vi "CANbus Mngr 1.vi"(5 "DBC File":path=path "C:/Users/ykouchnir/Desktop/Comemso BCS Tester/BCS24_CAN-MatrixV7_12.dbc", 6 "interface":refnum<k21>="CAN1", 7 "Action":T3, 8 "error in (no error)":errorcluster, 9 "Transfer Type":T1, 10 "database alias":string="Database", 11 "Data in":T2[](array[typedef])) -> (0 "error out":errorcluster, 3 "Data out":T2[](array[typedef]))   [LabVIEW 2021]
uses:
  <vilib>/xnet/xnet.llb/XNET Create Session (Signal Input Single-point).vi
  <resource>/objmgr/xnet.rc
  <vilib>/xnet/xnet.llb/XNET Read (Signal Single-point).vi
  <vilib>/xnet/xnet.llb/XNET Write (Frame CAN).vi
  <vilib>/xnet/xnet.llb/XNET Create Session (Frame Output Single-point).vi
  <vilib>/xnet/xnet.llb/XNET Write (Signal Single-point).vi
  <vilib>/xnet/xnet.llb/XNET Create Session (Conversion).vi
  <vilib>/xnet/xnet.llb/XNET Read (Frame CAN).vi
  <vilib>/xnet/xnet.llb/XNET Convert (Signal to Frame CAN).vi
  controls/Signal Data.ctl
  <vilib>/xnet/xnet.llb/XNET Create Session (Frame Input Single-point).vi
  <vilib>/xnet/xnet.llb/XNET Create Session (Signal Output Single-point).vi
  controls/BCS Manager.ctl
  controls/Transfer Type.ctl
panel:
  in  "JSON?":bool
  in  "JSON signals file":path
  in  "timeout":i32=-1
  in  "number to read":i32=-1
  in  "Termination":u32(ring) items=["Off", "On"]
  in  "Baud Rate":u64=1000000
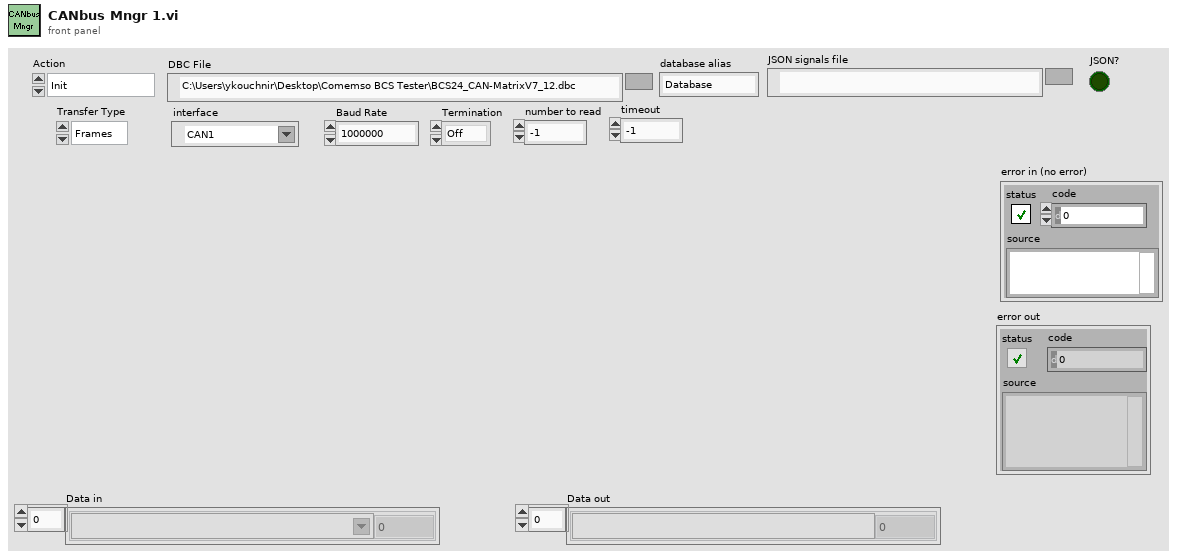
[diagram p1: front panel]
types:
  T1 = typedef "Transfer Type.ctl" = enum16{"Frames", "Signals"}
  T2 = typedef "Signal Data.ctl" = cluster{"XNET Signal":refnum<k21>, "Data":dbl}
  T3 = typedef "BCS Manager.ctl" = enum16{"Init", "Start Signal Session", "Start Frame Session", "Write Sigs Session", "Write Frames Session", "Write Sigs Single", "Write Frames Single", "Read Sigs Session", "Read Frames Session", "Read Sigs Single", "Read Frames Single", "Write Raw Frame Session", "Write Raw Frame Single", "FrameRef to Sigs", "FrameID to FrameRef", "Close"}
  T4 = typedef "JSON sigs.ctl" = cluster{"Read Signals Cyclic":refnum<k21>[], "Write Signals Cyclic":refnum<k21>[], "Write Frames Cyclic":refnum<k21>[], "Read Frames Cyclic":refnum<k21>[], "Write Frames Single":refnum<k21>[], "Read Frames Single":refnum<k21>[], "Write Signals Single":refnum<k21>[], "Read Signals Single":refnum<k21>[]}
  T5 = typedef "XNET Frame CAN.ctl" = cluster{"timestamp":timestamp, "payload":u8[], "identifier":u32, "type":T6, "extended?":bool, "echo?":bool}
  T6 = typedef "XNET Frame Type CAN.ctl" = u8
  T7 = typedef "Frame Data.ctl" = cluster{"Raw Frame":T5, "Frame Name":refnum<k21>, "Signals":T2[]}
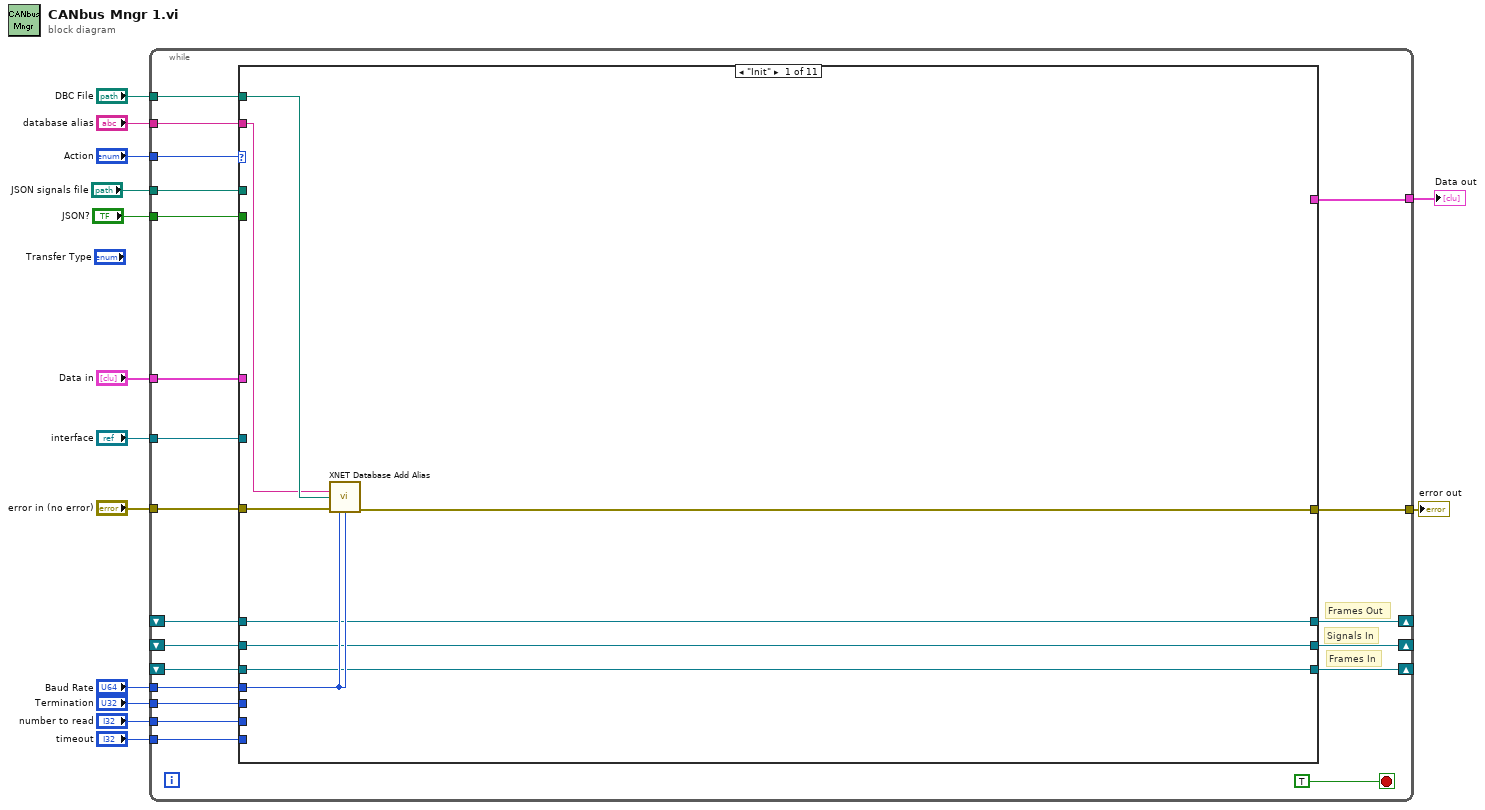
[diagram p0: block diagram]
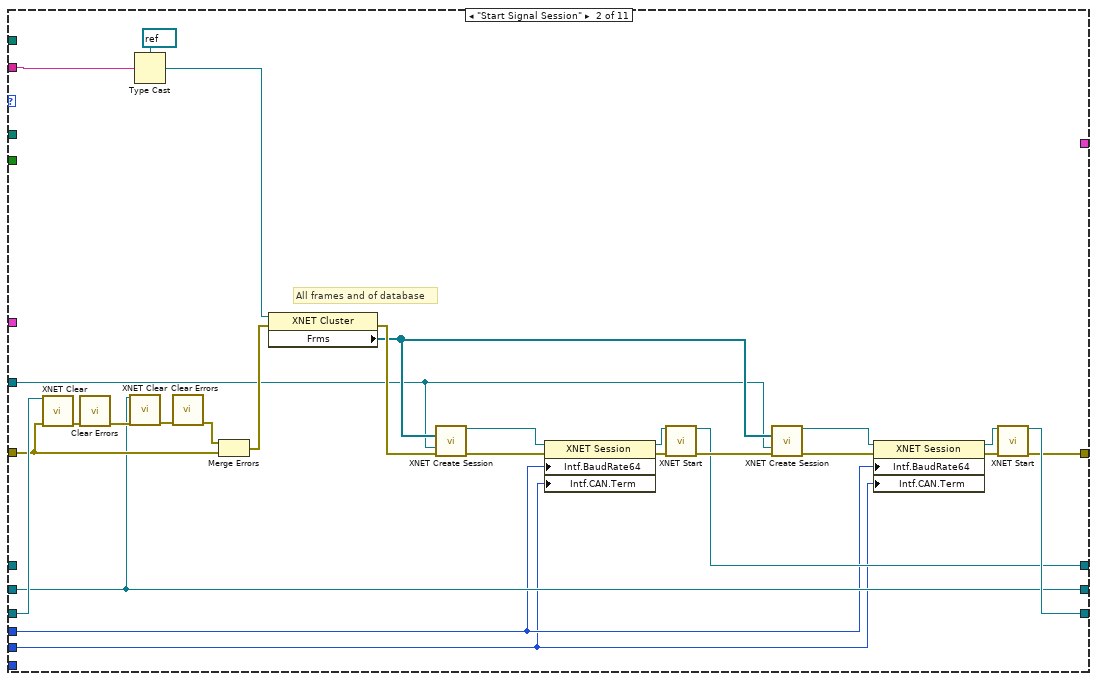
[diagram p2: hidden frame]
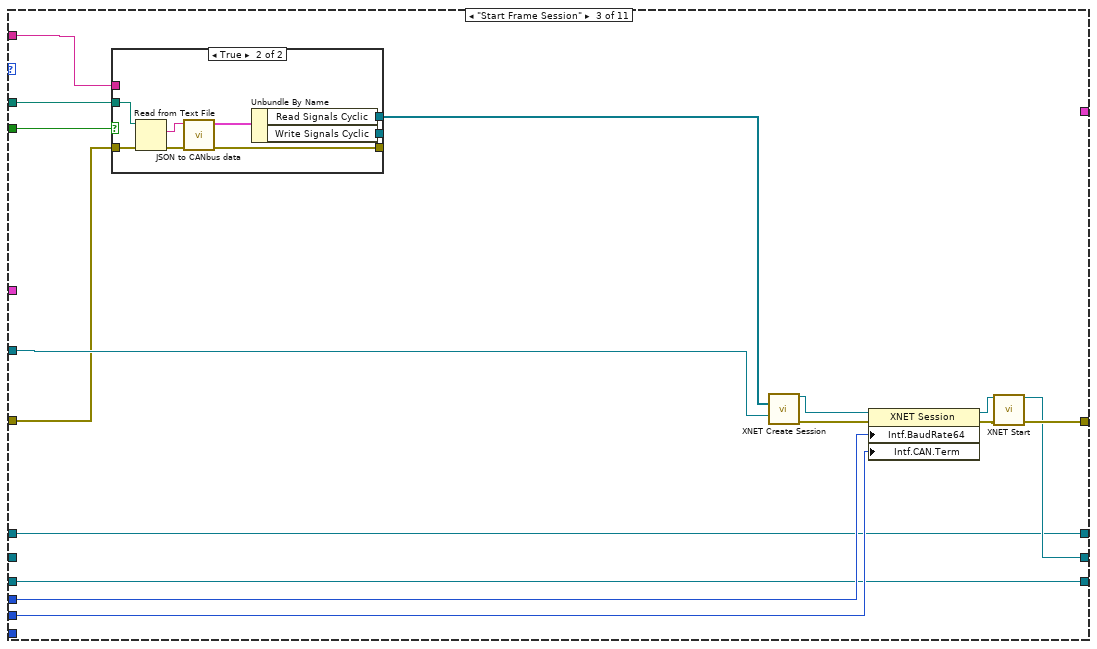
[diagram p3: hidden frame]
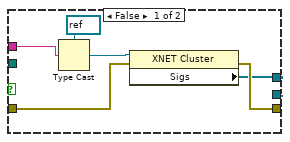
[diagram p4: hidden frame]
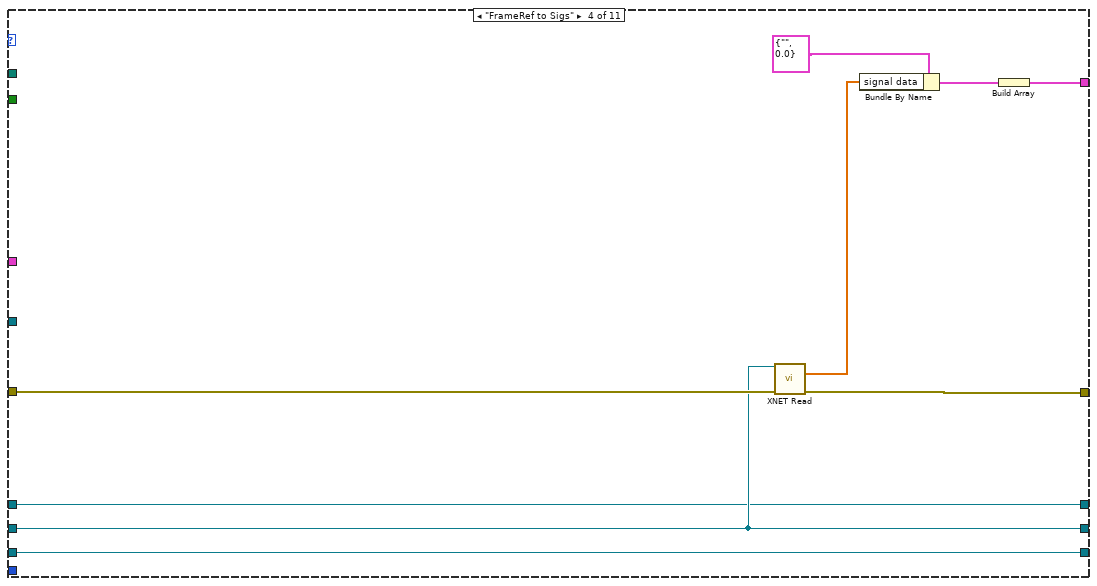
[diagram p5: hidden frame]
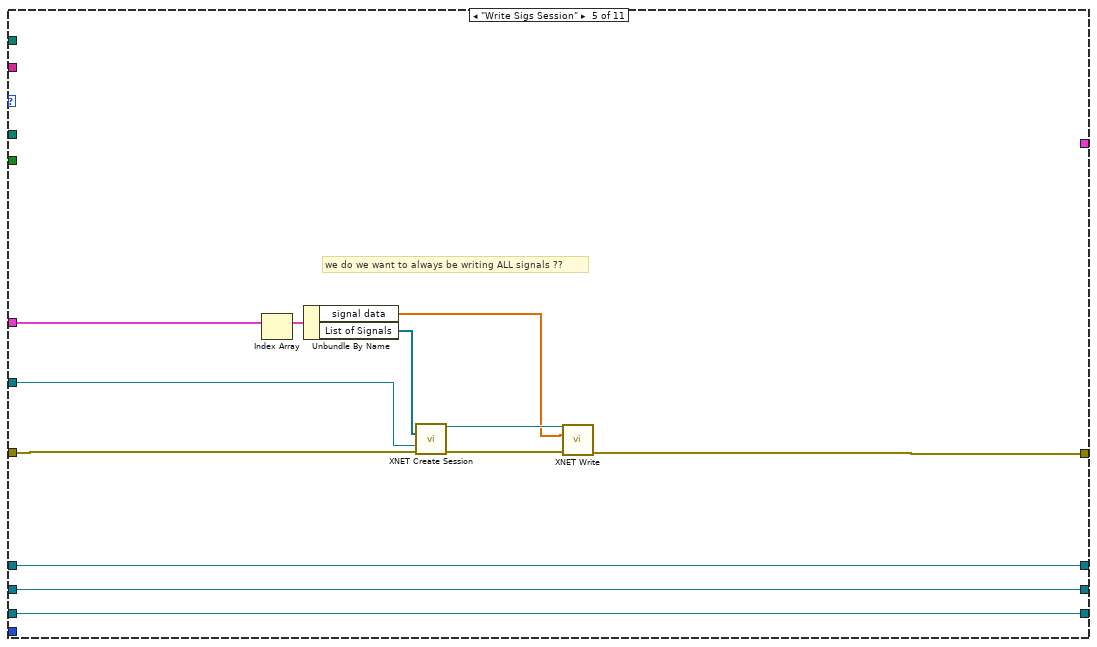
[diagram p6: hidden frame]
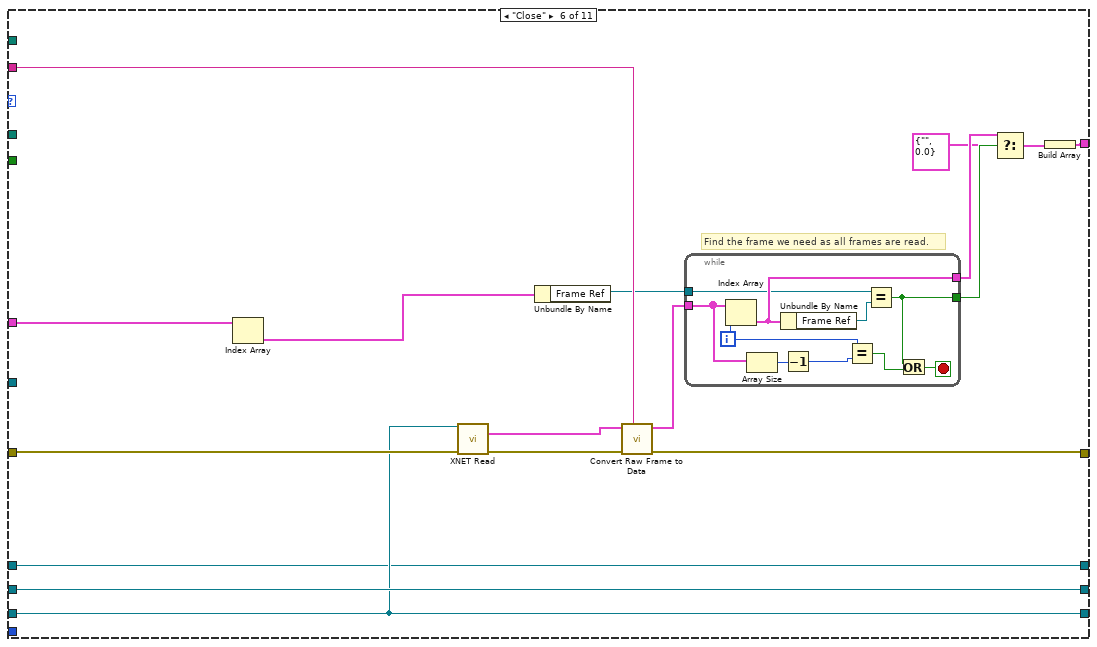
[diagram p7: hidden frame]
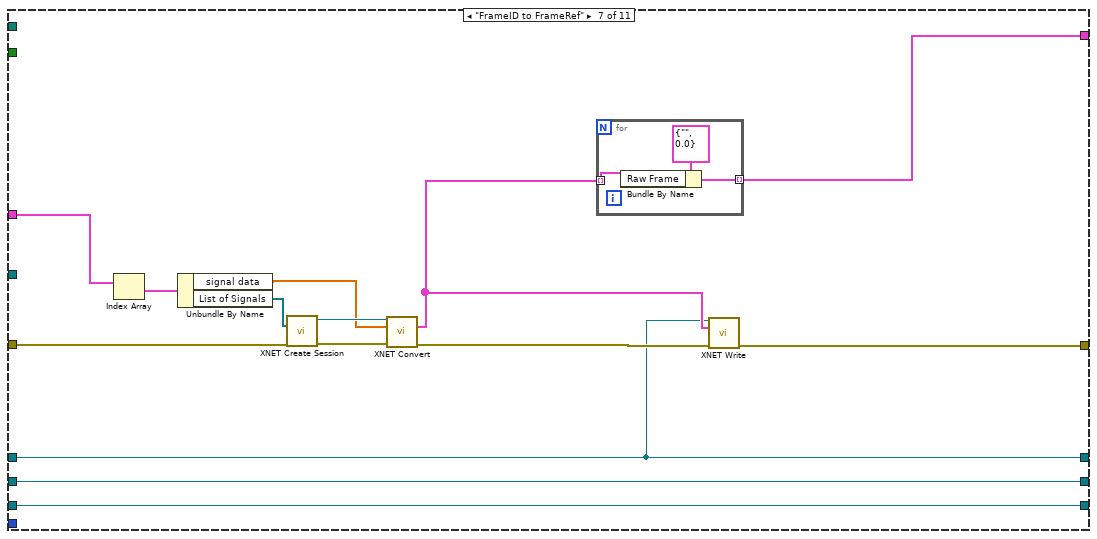
[diagram p8: hidden frame]
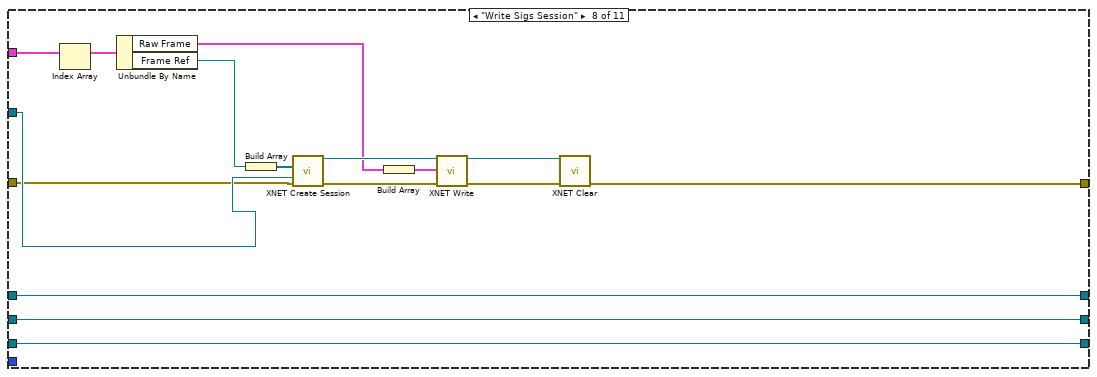
[diagram p9: hidden frame]
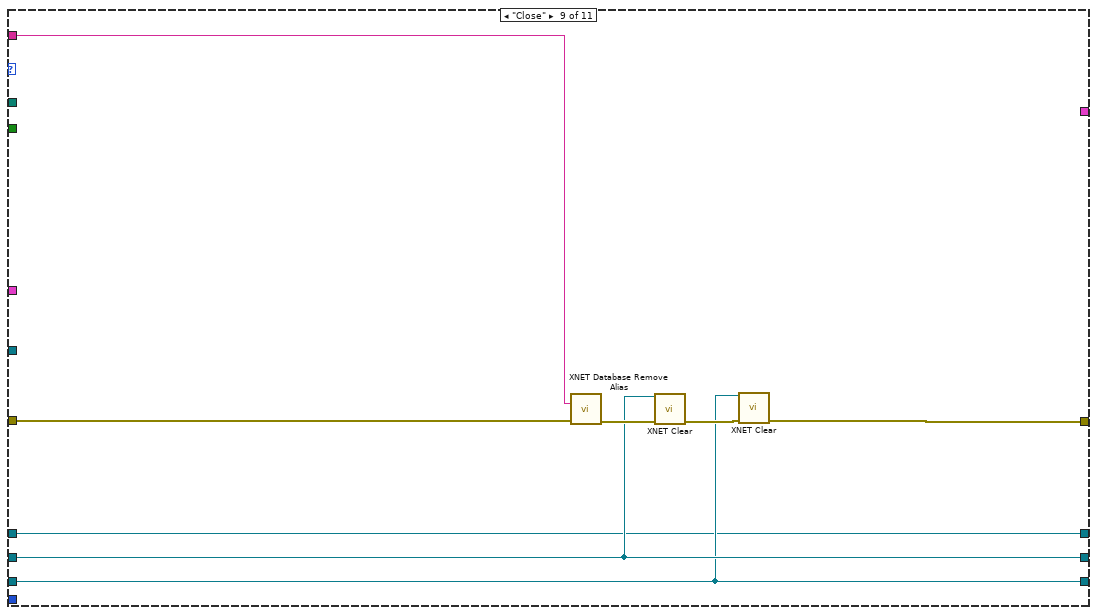
[diagram p10: hidden frame]
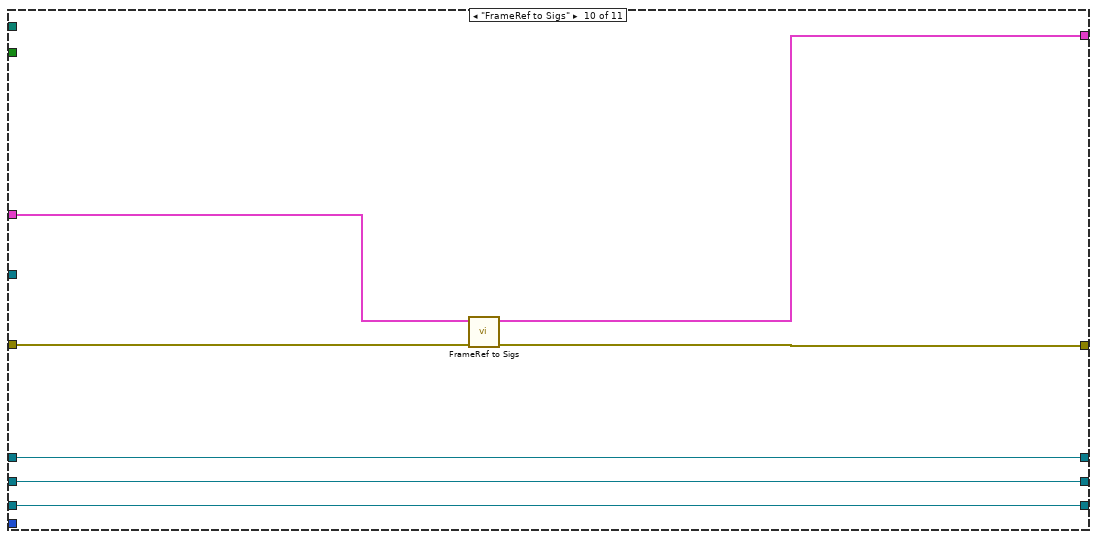
[diagram p11: hidden frame]
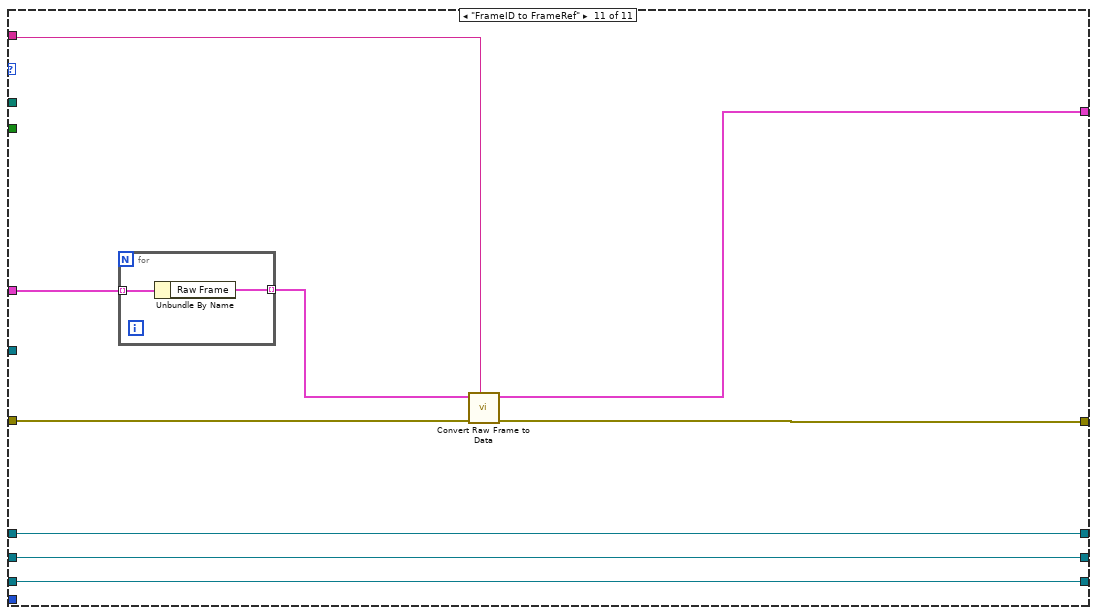
[diagram p12: hidden frame]
diagram:
  n1 = while {
    tunnel: "Action" -> [w34]
    tunnel: "error in (no error)" -> [w33]
    tunnel: "DBC File" -> [w32]
    tunnel: [w31] -> w11
    tunnel: "Baud Rate" -> [w30]
    tunnel: "Termination" -> [w29]
    tunnel: "interface" -> [w28]
    tunnel: "database alias" -> [w27]
    tunnel: [w19] -> w6
    tunnel: "Data in" -> [w26]
    tunnel: "number to read" -> [w25]
    tunnel: "timeout" -> [w24]
    shift-right: [w22] -> _
    shift-left: _ -> [w21]
    shift-right: [w23] -> _
    shift-left: _ -> [w20]
    tunnel: "JSON signals file" -> [w18]
    shift-right: [w16] -> _
    shift-left: _ -> [w17]
    tunnel: "JSON?" -> [w15]
    stop <- TRUE stop-if-true
    # "Frames Out"
    # "Frames In"
    # "Signals In"
    n2 = case shown="\"Init\"" w34 {
      tunnel: w33 -> [w43 w60 w73 w109 w122 w138 w163 w177 w190 w195 w204]
      tunnel: w32 -> [w42 _ _ _ _ _ _ _ _ _ _]
      tunnel: [w37 w63 w87 w110 w112 w139 w162 w172 w187 w194 w203] -> w31
      tunnel: w30 -> [w40 w45 w84 _ _ _ _ _ _ _ _]
      tunnel: w29 -> [_ w44 w85 _ _ _ _ _ _ _ _]
      tunnel: w28 -> [_ w52 w78 _ w121 _ _ w180 _ _ _]
      tunnel: w27 -> [w41 w71 w75 _ _ w135 _ _ w186 _ w202]
      tunnel: w26 -> [_ _ _ _ w116 w125 w157 w171 _ w193 w201]
      tunnel: w25 -> [_ _ _ _ _ _ _ _ _ _ _]
      tunnel: w24 -> [_ _ _ _ _ _ _ _ _ _ _]
      tunnel: [w38 w69 w77 w108 w119 w133 w160 w178 w184 w197 w206] -> w23
      tunnel: [w39 w58 w86 w105 w120 w134 w161 w179 w185 w196 w205] -> w22
      tunnel: w21 -> [w39 w58 _ w105 w120 w134 w161 w179 w185 w196 w205]
      tunnel: w20 -> [w38 w62 w77 w108 w119 w133 w160 w178 w184 w197 w206]
      tunnel: [_ _ _ w104 _ w126 w153 _ _ w192 w199] -> w19
      tunnel: w18 -> [_ _ w74 _ _ _ _ _ _ _ _]
      tunnel: [w36 w50 w72 w102 w111 w123 w150 w167 w183 w191 w198] -> w16
      tunnel: w17 -> [w36 _ w72 w102 w111 w123 w150 w167 w183 w191 w198]
      tunnel: w15 -> [_ _ w76 _ _ _ _ _ _ _ _]
      frame "Init" {
        n3 = call <vilib>:"XNET Database Add Alias.vi"("default baud rate (0)"=w40, "default FD baud rate (0)"=w40, "alias"=w41, "filepath"=w42, "error in (no error)"=w43) -> ("error out"=w37:errorcluster)  [unwired: 10 in]
      }
      frame "Start Signal Session" {
        # "All frames and of database"
        n4 = call <vilib>:"XNET Clear.vi"("session in"=w62, "error in (no error)"=w60) -> ("error out"=w61:errorcluster)  [unwired: 13 in]
        n5 = call <vilib>:"Clear Errors.vi"("error in (no error)"=w61) -> ("error out"=w59:errorcluster)  [unwired: 5 in, 1 out]
        n6 = call <vilib>:"XNET Clear.vi"("session in"=w58, "error in (no error)"=w59) -> ("error out"=w57:errorcluster)  [unwired: 13 in]
        n7 = Type Cast(type=refnum<k21> refnum ("cluster (:memory:)"), x=w71) -> (*(type *) &x=w68:refnum<k21>)
        n8 = call <vilib>:"Clear Errors.vi"("error in (no error)"=w57) -> ("error out"=w56:errorcluster)  [unwired: 5 in, 1 out]
        n9 = Merge Errors(w56, w60) -> (w55:errorcluster)
        n10 = property class="XNET Cluster"(reference=w68, error in=w55) -> (error out=w54:errorcluster, "Frms"=w53:refnum<k21>[])  [unwired: 1 out]
        n11 = call-poly <vilib>:"XNET Create Session.vi"("frame list"=w53, "interface"=w52, "error in (no error)"=w54) -> ("session out"=w47:refnum<k21>, "error out"=w49:errorcluster)  [unwired: 11 in]
        n12 = property class="XNET Session"(reference=w47, error in=w49, "Intf.BaudRate64"=w45, "Intf.CAN.Term"=w44) -> (reference out=w46:refnum<k21>, error out=w48:errorcluster)
        n13 = call <vilib>:"XNET Start.vi"("session in"=w46, "error in (no error)"=w48) -> ("session out"=w50:refnum<k21>, "error out"=w51:errorcluster)  [unwired: 12 in]
        n14 = call-poly <vilib>:"XNET Create Session.vi"("frame list"=w53, "interface"=w52, "error in (no error)"=w51) -> ("session out"=w67:refnum<k21>, "error out"=w65:errorcluster)  [unwired: 11 in]
        n15 = property class="XNET Session"(reference=w67, error in=w65, "Intf.BaudRate64"=w45, "Intf.CAN.Term"=w44) -> (reference out=w66:refnum<k21>, error out=w64:errorcluster)
        n16 = call <vilib>:"XNET Start.vi"("session in"=w66, "error in (no error)"=w64) -> ("session out"=w69:refnum<k21>, "error out"=w63:errorcluster)  [unwired: 12 in]
      }
      frame "Start Frame Session" {
        n17 = case shown="True" w76 {
          tunnel: w75 -> [w89 _]
          tunnel: [w92 w98] -> w83
          tunnel: [w93 w99] -> _
          tunnel: [w92 w97] -> _
          tunnel: w74 -> [_ w96]
          tunnel: w73 -> [w88 w95]
          frame False {
            n18 = Type Cast(type=refnum<k21> refnum ("cluster (:memory:)"), x=w89) -> (*(type *) &x=w90:refnum<k21>)
            n19 = property class="XNET Cluster"(reference=w90, error in=w88) -> (error out=w93:errorcluster, "Sigs"=w92:refnum<k21>[])  [unwired: 1 out]
          }
          frame True {
            n20 = Read from Text File(file (use dialog)=w96, error in=w95) -> (text=w100:string, error out=w101:errorcluster)  [unwired: 2 in, 2 out]
            n21 = call "JSON to CANbus data.vi"("error in"=w101, "JSON string"=w100) -> ("error out"=w99:errorcluster, "Signal Sessions"=w94:T4)  [unwired: 8 in]
            n22 = Unbundle By Name(w94) -> ("Read Signals Cyclic"=w98:refnum<k21>[], "Write Signals Cyclic"=w97:refnum<k21>[])
          }
        }
        n23 = call-poly <vilib>:"XNET Create Session.vi"("signal list"=w83, "interface"=w78) -> ("session out"=w82:refnum<k21>, "error out"=w80:errorcluster)  [unwired: 12 in]
        n24 = property class="XNET Session"(reference=w82, error in=w80, "Intf.BaudRate64"=w84, "Intf.CAN.Term"=w85) -> (reference out=w81:refnum<k21>, error out=w79:errorcluster)
        n25 = call <vilib>:"XNET Start.vi"("session in"=w81, "error in (no error)"=w79) -> ("session out"=w86:refnum<k21>, "error out"=w87:errorcluster)  [unwired: 12 in]
      }
      frame "FrameRef to Sigs" {
        n26 = call-poly <vilib>:"XNET Read.vi"("session in"=w105, "error in (no error)"=w109) -> ("data"=w107:dbl[], "error out"=w110:errorcluster)  [unwired: 11 in, 1 out]
        n27 = Bundle By Name(cluster=T2 {"XNET Signal"="", "Data"=0.0} ("Data out"), "signal data"=w107) -> (w106:T2)
        n28 = Build Array(w106) -> (w104:T2[])
      }
      frame "Write Sigs Session" {
        # "we do we want to always be writing ALL signals ??"
        n29 = Index Array(array=w116) -> (element=w115:T2)  [unwired: 1 in]
        n30 = Unbundle By Name(w115) -> ("signal data"=w113:dbl[], "List of Signals"=w114:refnum<k21>[])
        n31 = call-poly <vilib>:"XNET Create Session.vi"("signal list"=w114, "interface"=w121, "error in (no error)"=w122) -> ("session out"=w118:refnum<k21>, "error out"=w117:errorcluster)  [unwired: 11 in]
        n32 = call-poly <vilib>:"XNET Write.vi"("session in"=w118, "data"=w113, "error in (no error)"=w117) -> ("error out"=w112:errorcluster)  [unwired: 11 in, 1 out]
      }
      frame "Close" {
        # "Find the frame we need as all frames are read."
        n33 = Index Array(array=w125) -> (element=w124:T2)  [unwired: 1 in]
        n34 = call-poly <vilib>:"XNET Read.vi"("session in"=w133, "error in (no error)"=w138) -> ("data"=w136:T5[], "error out"=w137:errorcluster)  [unwired: 10 in, 2 out]
        n35 = Unbundle By Name(w124) -> ("Frame Ref"=w131:refnum<k21>)
        n36 = call "Convert Raw Frame to Data.vi"("Database alias"=w135, "error in (no error)"=w137, "Raw Frames"=w136) -> ("error out"=w139:errorcluster, "Frame Data"=w132:T7[])  [unwired: 7 in]
        n37 = while {
          tunnel: w132 -> [w148]
          tunnel: w131 -> [w140]
          tunnel: [w142] -> w129
          tunnel: [w141] -> w130
          i -> [w146]
          stop <- w143 stop-if-true
          n38 = Index Array(array=w148, index=w146) -> (element=w142:T7)
          n39 = Array Size(array=w148) -> (size(s)=w147:i32)
          n40 = Unbundle By Name(w142) -> ("Frame Ref"=w149:refnum<k21>)
          n41 = Decrement(x=w147) -> (x-1=w145:i32)
          n42 = Equal?(x=w146, y=w145) -> (x = y?=w144:bool)
          n43 = Equal?(x=w140, y=w149) -> (x = y?=w141:bool)
          n44 = Or(x=w141, y=w144) -> (x .or. y?=w143:bool)
        }
        n45 = Select(t=w129, s=w130, f=T2 {"XNET Signal"="", "Data"=0.0}) -> (s? t:f=w127:T7)
        n46 = Build Array(w127) -> (w126:T7[])
      }
      frame "FrameID to FrameRef" {
        n47 = Index Array(array=w157) -> (element=w156:T2)  [unwired: 1 in]
        n48 = Unbundle By Name(w156) -> ("signal data"=w155:dbl[], "List of Signals"=w154:refnum<k21>[])
        n49 = call-poly <vilib>:"XNET Create Session.vi"("signal list"=w154, "error in (no error)"=w163) -> ("session out"=w158:refnum<k21>, "error out"=w159:errorcluster)  [unwired: 12 in]
        n50 = call-poly <vilib>:"XNET Convert.vi"("session in"=w158, "signal data"=w155, "error in (no error)"=w159) -> ("frame data"=w152:T5[], "error out"=w151:errorcluster)  [unwired: 9 in, 2 out]
        n51 = for {
          tunnel: w152 -> [w165] mode=indexing
          tunnel: [w164] -> w153 mode=indexing
          n52 = Bundle By Name(cluster=T2 {"XNET Signal"="", "Data"=0.0} ("f"), "Raw Frame"=w165) -> (w164:T2)
        }
        n53 = call-poly <vilib>:"XNET Write.vi"("session in"=w150, "data"=w152, "error in (no error)"=w151) -> ("error out"=w162:errorcluster)  [unwired: 11 in, 1 out]
      }
      frame "Write Sigs Session" {
        n54 = Index Array(array=w171) -> (element=w170:T2)  [unwired: 1 in]
        n55 = Unbundle By Name(w170) -> ("Raw Frame"=w176:T5, "Frame Ref"=w175:refnum<k21>)
        n56 = Build Array(w175) -> (w169:refnum<k21>[])
        n57 = call-poly <vilib>:"XNET Create Session.vi"("frame list"=w169, "interface"=w180, "error in (no error)"=w177) -> ("session out"=w181:refnum<k21>, "error out"=w182:errorcluster)  [unwired: 11 in]
        n58 = Build Array(w176) -> (w168:T5[])
        n59 = call-poly <vilib>:"XNET Write.vi"("session in"=w181, "data"=w168, "error in (no error)"=w182) -> ("session out"=w173:refnum<k21>, "error out"=w174:errorcluster)  [unwired: 11 in]
        n60 = call <vilib>:"XNET Clear.vi"("session in"=w173, "error in (no error)"=w174) -> ("error out"=w172:errorcluster)  [unwired: 13 in]
      }
      frame "Close" {
        n61 = call <vilib>:"XNET Database Remove Alias.vi"("alias"=w186, "error in (no error)"=w190) -> ("error out"=w189:errorcluster)  [unwired: 13 in]
        n62 = call <vilib>:"XNET Clear.vi"("session in"=w185, "error in (no error)"=w189) -> ("error out"=w188:errorcluster)  [unwired: 13 in]
        n63 = call <vilib>:"XNET Clear.vi"("session in"=w184, "error in (no error)"=w188) -> ("error out"=w187:errorcluster)  [unwired: 13 in]
      }
      frame "FrameRef to Sigs" {
        n64 = call "FrameRef to Sigs.vi"("error in (no error)"=w195, "Data in"=w193) -> ("error out"=w194:errorcluster, "Signals"=w192:T2[])  [unwired: 8 in]
      }
      frame "FrameID to FrameRef" {
        n65 = for {
          tunnel: [w208] -> w200 mode=indexing
          tunnel: w201 -> [w207] mode=indexing
          n66 = Unbundle By Name(w207) -> ("Raw Frame"=w208:T5)
        }
        n67 = call "Convert Raw Frame to Data.vi"("Database alias"=w202, "error in (no error)"=w204, "Raw Frames"=w200) -> ("error out"=w203:errorcluster, "Frame Data"=w199:T7[])  [unwired: 7 in]
      }
    }
  }
  "error out" <- w11
  "Data out" <- w6
